vi "AutoShoot.vi"() -> (0 "Terminate":bool)   [LabVIEW 2015]
uses:
  Utilities/AutoShootControl.ctl
  <vilib>/Rock Robotics/WPI/Solenoid/WPI_SolenoidValue.ctl
  Utilities/MotorPositionGlobals.vi
  <vilib>/Rock Robotics/WPI/Solenoid/WPI_SolenoidSetEnum.vi
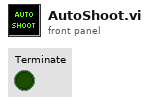
[diagram p1: front panel]
types:
  T1 = typedef "AutoShootControl.ctl" = enum16{"SetShot", "Shoot", "Reload", "Release"}
  T2 = typedef "WPI_SolenoidDevRef.ctl" = cluster{"DevStatus":errorcluster, "Pneumatics Control Module":u8, "Forward Solenoid Channel":T3, "Reverse Solenoid Channel":T3}
  T3 = typedef "WPI_SolenoidChannel.ctl" = enum8{"Solenoid 0", "Solenoid 1", "Solenoid 2", "Solenoid 3", "Solenoid 4", "Solenoid 5", "Solenoid 6", "Solenoid 7", "Invalid"}
  T4 = typedef "WPI_SolenoidValue.ctl" = enum16{"Off", "On", "Forward", "Reverse"}
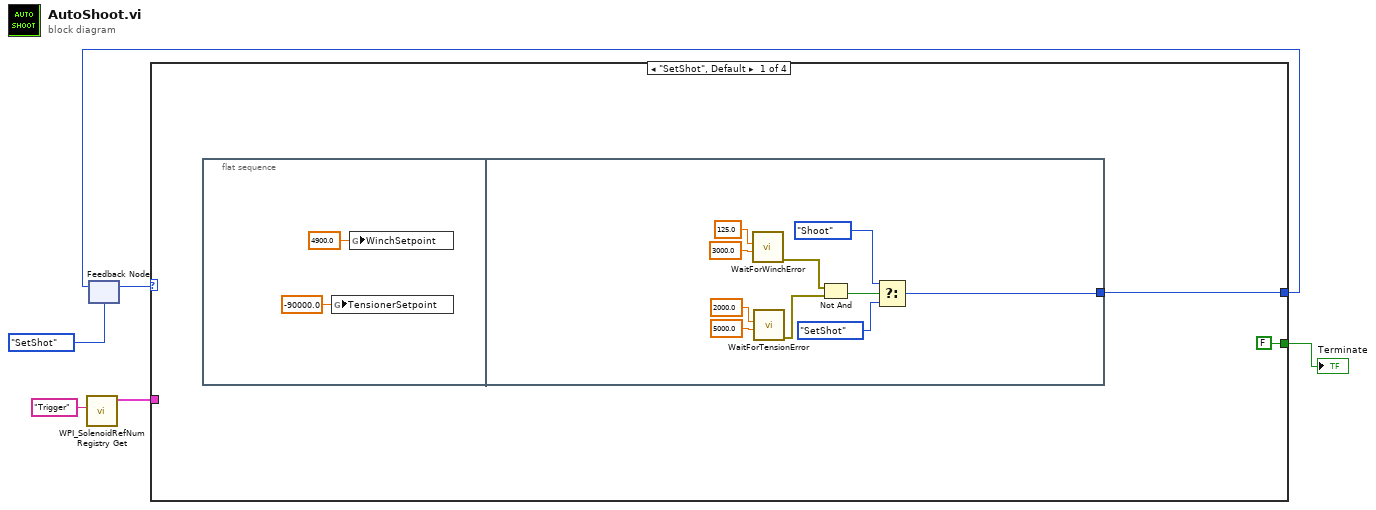
[diagram p0: block diagram]
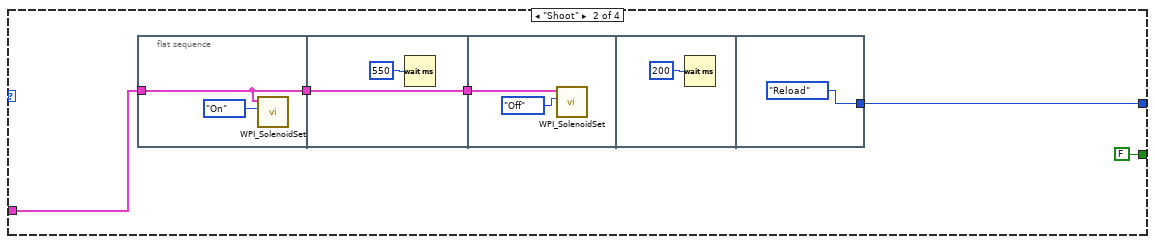
[diagram p2: hidden frame]
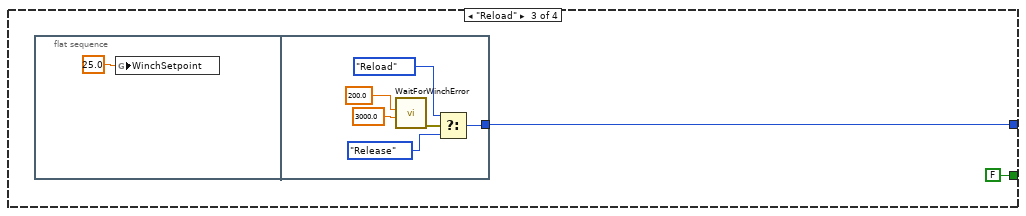
[diagram p3: hidden frame]
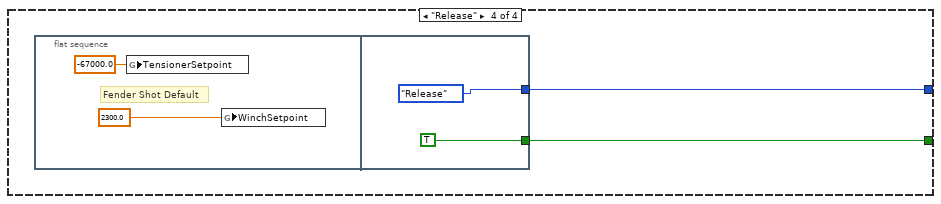
[diagram p4: hidden frame]
diagram:
  n1 = call <vilib>:"WPI_SolenoidRefNum Registry Get.vi"("refnum name"="Trigger") -> ("SolenoidDevRef"=w2:T2)  [unwired: 9 in, 1 out]
  n2 = feedback #1(AutoShootControl."SetShot" ("Enum")) -> (w5:T1)
  n3 = case shown="\"SetShot\", Default" w5 {
    tunnel: [w8 w22 w35 w44] -> w4
    tunnel: w2 -> [_ w23 _ _]
    tunnel: [FALSE FALSE FALSE w43] -> w1
    frame "SetShot", Default {
      n4 = flat-sequence {
        tunnel: [w11] -> w8
        frame #0 {
          n5 = global write "MotorPositionGlobals.vi" "TensionerSetpoint"(-90000.0 ("TensionerSetpoint")) -> ()
          n6 = global write "MotorPositionGlobals.vi" "WinchSetpoint"(4900.0 ("WinchSetpoint")) -> ()
        }
        frame #1 {
          n7 = call "WaitForWinchError.vi"("Timeout (ms)"=3000.0, "AllowedError"=125.0) -> ("error out"=w15:errorcluster)  [unwired: 9 in]
          n8 = call "WaitForTensionError.vi"("Timeout (ms)"=5000.0, "AllowedError"=2000.0) -> ("error out"=w16:errorcluster)  [unwired: 9 in]
          n9 = Not And(1:w16, 2:w15) -> (0:w14:bool)
          n10 = Select(t=AutoShootControl."Shoot" ("Enum"), s=w14, f=AutoShootControl."SetShot" ("Enum")) -> (s? t:f=w11:T1)
        }
      }
    }
    frame "Shoot" {
      n11 = flat-sequence {
        tunnel: w23 -> [w26]
        tunnel: [w26] -> w25
        tunnel: w25 -> [w28]
        tunnel: [w28] -> w24
        tunnel: w24 -> [w30]
        tunnel: [AutoShootControl."Reload" ("Enum")] -> w22
        frame #0 {
          n12 = call-poly <vilib>:"WPI_SolenoidSet.vi"("Value"=WPI_SolenoidValue."On", "SolenoidDevRef"=w26) -> ()  [unwired: 8 in, 2 out]
        }
        frame #1 {
          n13 = Wait (ms)(milliseconds to wait=u32 550) -> ()  [unwired: 1 out]
        }
        frame #2 {
          n14 = call-poly <vilib>:"WPI_SolenoidSet.vi"("Value"=WPI_SolenoidValue."Off", "SolenoidDevRef"=w30) -> ()  [unwired: 8 in, 2 out]
        }
        frame #3 {
          n15 = Wait (ms)(milliseconds to wait=u32 200) -> ()  [unwired: 1 out]
        }
        frame #4 {
        }
      }
    }
    frame "Reload" {
      n16 = flat-sequence {
        tunnel: [w39] -> w35
        frame #0 {
          n17 = global write "MotorPositionGlobals.vi" "WinchSetpoint"(25.0 ("WinchPosition")) -> ()
        }
        frame #1 {
          n18 = call "WaitForWinchError.vi"("Timeout (ms)"=3000.0, "AllowedError"=200.0) -> ("error out"=w40:errorcluster)  [unwired: 9 in]
          n19 = Select(t=AutoShootControl."Reload" ("Enum"), s=w40, f=AutoShootControl."Release" ("Enum")) -> (s? t:f=w39:T1)
        }
      }
    }
    frame "Release" {
      n20 = flat-sequence {
        tunnel: [AutoShootControl."Release" ("Enum")] -> w44
        tunnel: [TRUE] -> w43
        frame #0 {
          # "Fender Shot Default"
          n21 = global write "MotorPositionGlobals.vi" "TensionerSetpoint"(-67000.0 ("TensionerSetpoint")) -> ()
          n22 = global write "MotorPositionGlobals.vi" "WinchSetpoint"(2300.0 ("WinchPosition")) -> ()
        }
        frame #1 {
        }
      }
    }
  }
  "Terminate" <- w1
  n23 = feedback-in #1(w4) -> ()
